vi "Make from Test Case.vi"(8 "error in (no error)":errorcluster, 10 "LUnit Test Case":refnum<class "LUnit Test Case.lvclass">) -> (0 "error out":errorcluster, 3 "LUnit Test Suite Out":refnum<class "LUnit Test Suite.lvclass">)   [LabVIEW 2020, in "LUnit Test Suite.lvclass"]
uses:
  LUnit Test Suite.lvclass
  LUnit Test Case/LUnit Test Case.lvclass
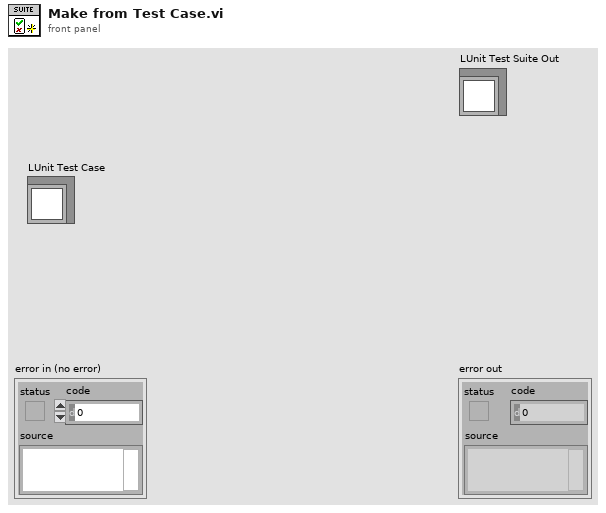
[diagram p1: front panel]
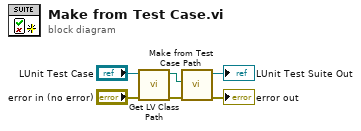
[diagram p0: block diagram]
diagram:
  n1 = call <vilib>:"Get LV Class Path.vi"("error in (no error)"="error in (no error)", "object"="LUnit Test Case") -> ("error out"=w3:errorcluster, "class path"=w4:path)  [unwired: 8 in]
  n2 = call "Make from Test Case Path.vi"("error in (no error)"=w3, "Test Case"=w4) -> ("error out"=→"error out":errorcluster, "LUnit Test Suite Out"=→"LUnit Test Suite Out":refnum<class "LUnit Test Suite.lvclass">)  [unwired: 8 in]
